vi "RT Driver VI.vi"(7 "Operation":T1, 11 "Device Reference in":T2 format="%.0x") -> (0 "Error Code":i32)   [LabVIEW 2021, in "Large Number Operation Engine.lvlib"]
uses:
  Large Number Operation Engine.lvlib
  <vilib>/NI VeriStand/Custom Device API/Custom Device Item Ref.ctl
  <vilib>/NI VeriStand/Custom Device API/Hardware Interface Driver VI Operation.ctl
  Shared/Compiled.Settings.ctl
  RTStateVariables.ctl
  <vilib>/NI/NIVS Inline Async API/_VS Inline Async API/VS Inline Async API/VS Inline Async API.lvclass
  <vilib>/NI/NIVS Inline Async API/_VS Inline Async API/VS Inline Async API/VS Inline Async API.lvclass/VS Inline Async API.ctl
  <vilib>/NI/NIVS Inline Async API/_Data Access Engine/Data Access Engine/Data Access Engine.lvclass/Data Access Engine.ctl
  <vilib>/NI/NIVS Inline Async API/_Data Access Engine/Access Type Classes/Write/Write.lvclass/Write.ctl
  <vilib>/NI/NIVS Inline Async API/_Data Access Engine/Access Type Classes/ReadWrite/ReadWrite.lvclass/ReadWrite.ctl
  <vilib>/NI/NIVS Inline Async API/_Data Access Engine/Access Type Classes/Read/Read.lvclass/Read.ctl
  <vilib>/NI/NIVS Inline Async API/_Data Access Engine/Data Access Engine/Methods/Data.Engine.Read Data from HW.vi
  <vilib>/NI/NIVS Inline Async API/_VS Inline Async API/Error Handling Process/SubVIs/Error.GetError.vi
  <vilib>/NI/NIVS Inline Async API/_Data Access Engine/Data Access Engine/Methods/Data.Engine.Write Data to HW.vi
  <vilib>/NI/NIVS Inline Async API/_Data Access Engine/Access Type Classes/ReadWrite/ReadWrite.EngineData.vi
  <vilib>/NI/NIVS Inline Async API/_Data Access Engine/Access Type Classes/Write/Write.EngineData.vi
  <vilib>/NI/NIVS Inline Async API/_Data Access Engine/Access Type Classes/Read/Read.EngineData.vi
  <vilib>/NI VeriStand/Custom Device API/NI VeriStand - Get Channel Value by Data Reference.vi
  <vilib>/NI VeriStand/Custom Device API/NI VeriStand - Set Channel Value by Data Reference.vi
  <vilib>/NI VeriStand/Custom Device API/NI VeriStand - Get Channel Values by Block Data Reference.vi
  Large Number Operation.Async.vi
  Shared/Constants.vi
  <vilib>/NI VeriStand/Custom Device API/Get Item Property (Variant).vi
  <vilib>/NI VeriStand/Custom Device API/Global Data Refs.vi
  <vilib>/NI VeriStand/Custom Device API/Custom Device API.lvlib
  Shared/Large Number Operation Shared.lvlib
  <vilib>/NI VeriStand/Custom Device Tools/Custom Device Utility Library/Custom Device Utility Library.lvlib
panel:
  out "appended array":cluster{"VI":refnum<vi>, "Parameters":variant}[](array[cluster])
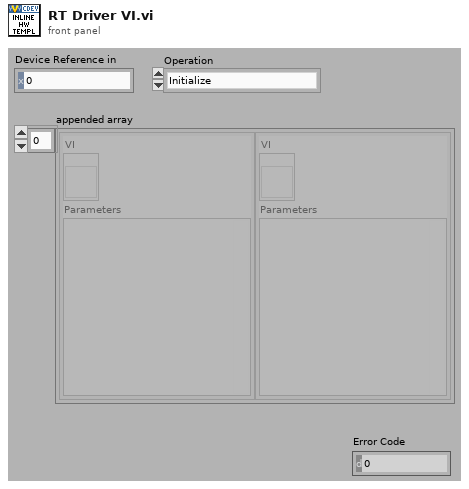
[diagram p1: front panel]
types:
  T1 = typedef "Custom Device API.lvlib/Hardware Interface Driver VI Operation.ctl" = enum16{"Initialize", "Start", "Read Data from HW", "Write Data to HW", "Close"}
  T2 = typedef "Custom Device API.lvlib/Custom Device Item Ref.ctl" = u64
  T3 = typedef "Large Number Operation Engine.lvlib/RTStateVariables.ctl" = cluster{"Async":refnum<class "VS Inline Async API.lvclass">, "Settings":T4}
  T4 = typedef "Large Number Operation Shared.lvlib/Compiled.Settings.ctl" = cluster{"Name":string, "Async Init Timeout":u16, "Address":string}
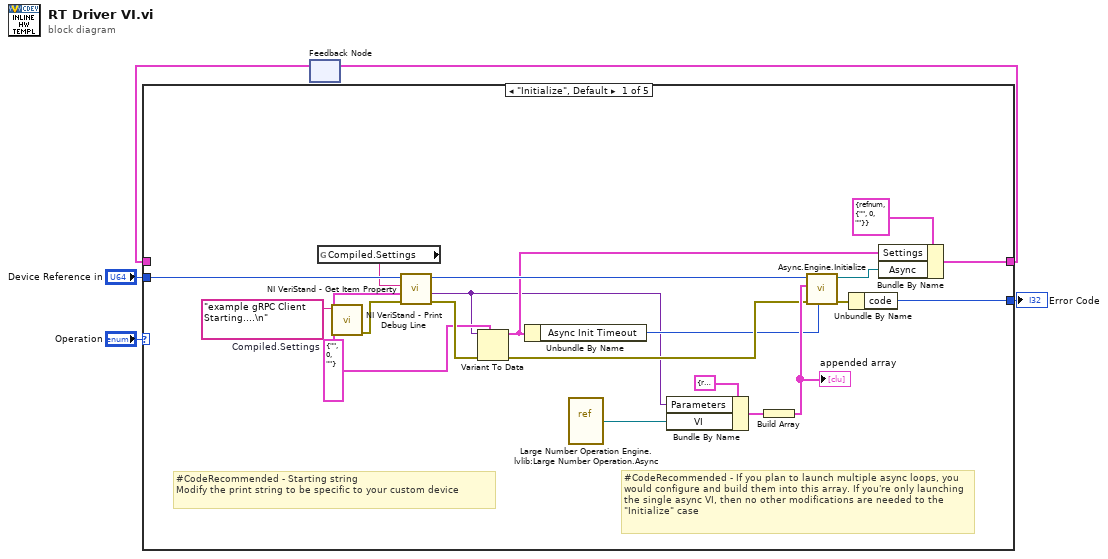
[diagram p0: block diagram]
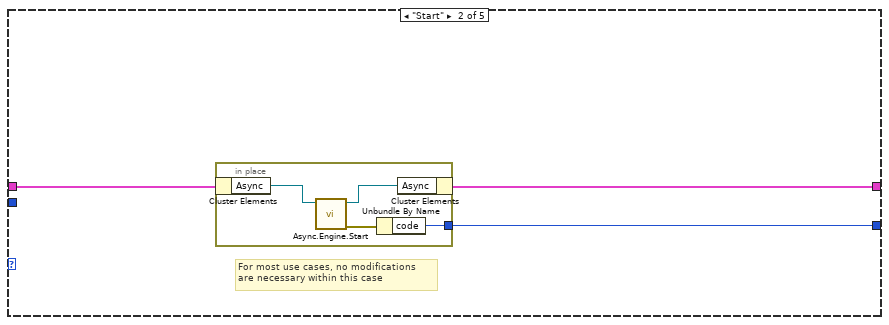
[diagram p2: hidden frame]
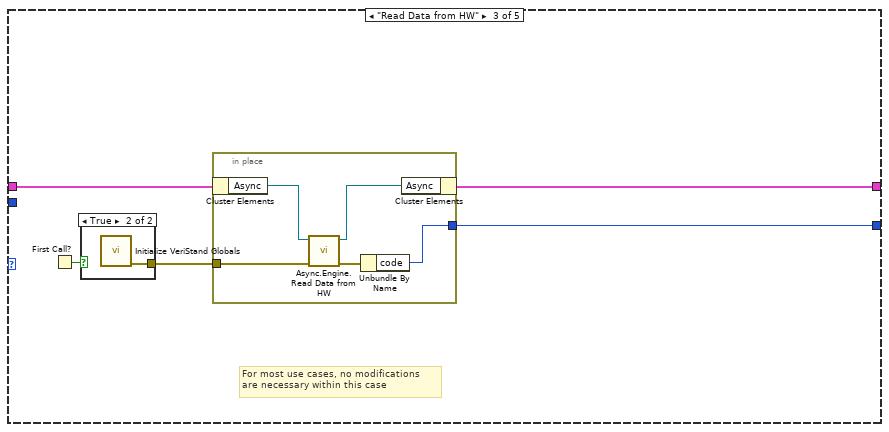
[diagram p3: hidden frame]
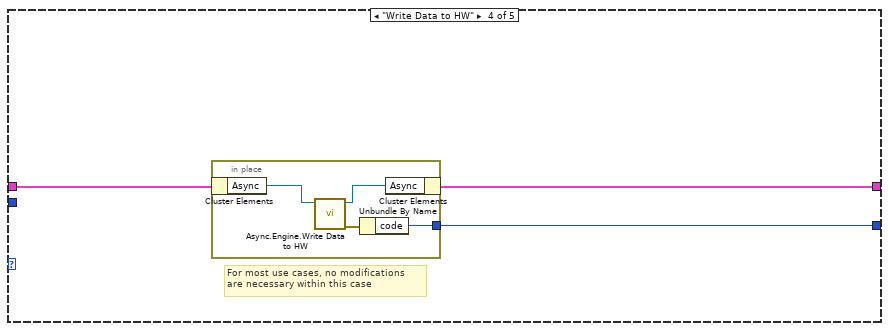
[diagram p5: hidden frame]
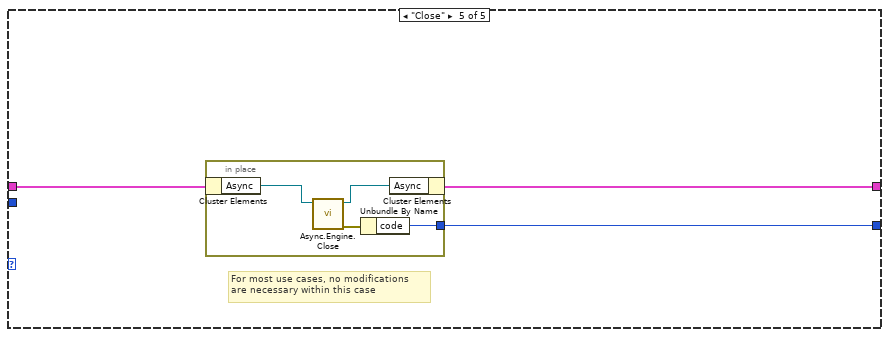
[diagram p6: hidden frame]
diagram:
  n1 = feedback #1() -> (w3:T3)  [unwired: 1 out]
  n2 = case shown="\"Initialize\", Default" "Operation" {
    tunnel: [w23 w27 w35 w44 w52] -> w4
    tunnel: w3 -> [_ w28 w37 w45 w53]
    tunnel: "Device Reference in" -> [w20 _ _ _ _]
    tunnel: [w25 w26 w36 w46 w51] -> w1
    frame "Initialize", Default {
      w16 = T4 {"Name"="", "Async Init Timeout"=0, "Address"=""}  # Compiled.Settings
      # "#CodeRecommended - Starting string\nModify the print string to be specific to your custom device"
      # "#CodeRecommended - If you plan to launch multiple async loops, you would configure and build them into this array. If you're only launching the single async VI, then no other modifications are needed to the \"Initialize\" case"
      n3 = global read "Constants.vi" "Compiled.Settings"() -> (w18:string)
      n4 = call <vilib>:"NI VeriStand - Print Debug Line.vi"("Message"="example gRPC Client Starting....\n") -> ("error out"=w12:errorcluster)  [unwired: 10 in]
      n5 = call-poly <vilib>:"NI VeriStand - Get Item Property.vi"("error in (no error)"=w12, "Default Value"=w16, "Property Name"=w18, "Item Ref in"=w20) -> ("error out"=w19:errorcluster, "Value"=w7:variant, "Item Ref out"=w13:T2)  [unwired: 4 in, 1 out]
      n6 = Variant To Data(error in=w19, type=w16, Variant=w7) -> (data=w8:T4, error out=w14:errorcluster)
      n7 = Unbundle By Name(w8) -> ("Async Init Timeout"=w9:u16)
      n8 = vi-ref "Large Number Operation Engine.lvlib:Large Number Operation.Async.vi"() -> (w10:refnum<vi>)
      n9 = Bundle By Name(cluster=cluster{"VI":refnum<vi>, "Parameters":variant} {"VI"=refnum, "Parameters"=variant} ("Process"), "Parameters"=w7, "VI"=w10) -> (w21:cluster{"VI":refnum<vi>, "Parameters":variant})
      n10 = Build Array(w21) -> (w15:cluster{"VI":refnum<vi>, "Parameters":variant}[])
      "appended array" <- w15
      n11 = call <vilib>:"Async.Engine.Initialize.vi"("Timeout (ms) (5000)"=w9, "error in (no error)"=w14, "Processes"=w15, "Custom Device Ref"=w13) -> ("error out"=w17:errorcluster, "Async"=w24:refnum<class "VS Inline Async API.lvclass">)  [unwired: 6 in]
      n12 = Unbundle By Name(w17) -> ("code"=w25:i32)
      n13 = Bundle By Name(cluster=T3 {"Async"=refnum, "Settings"={"Name"="", "Async Init Timeout"=0, "Address"=""}} ("RT State Variables"), "Settings"=w8, "Async"=w24) -> (w23:T3)
    }
    frame "Start" {
      # "For most use cases, no modifications \nare necessary within this case"
      n14 = in-place {
        in-place-border: [w29] -> w26
        n15 = in-place-cluster #2(w28) -> ("Async"=w32:refnum<class "VS Inline Async API.lvclass">)
        n16 = call <vilib>:"Async.Engine.Start.vi"("VS Inline Async API in"=w32) -> ("error out"=w30:errorcluster, "VS Inline Async API out"=w31:refnum<class "VS Inline Async API.lvclass">)  [unwired: 9 in]
        n17 = Unbundle By Name(w30) -> ("code"=w29:i32)
        n18 = in-place-cluster #2("Async"=w31) -> (w27:T3)
      }
    }
    frame "Read Data from HW" {
      # "For most use cases, no modifications \nare necessary within this case"
      n19 = First Call?() -> (First Call?: T/F=w33:bool)
      n20 = case shown="True" w33 {
        tunnel: [_ w38] -> w34
        frame False {
        }
        frame True {
          n21 = call "Initialize VeriStand Globals.vi"() -> ("error out"=w38:errorcluster)  [unwired: 11 in]
        }
      }
      n22 = in-place {
        in-place-border: [w41] -> w36
        in-place-border: w34 -> [w39]
        n23 = in-place-cluster #3(w37) -> ("Async"=w43:refnum<class "VS Inline Async API.lvclass">)
        n24 = call <vilib>:"Async.Engine.Read Data from HW.vi"("error in"=w39, "Async in"=w43) -> ("error out"=w40:errorcluster, "Async out"=w42:refnum<class "VS Inline Async API.lvclass">)  [unwired: 8 in]
        n25 = Unbundle By Name(w40) -> ("code"=w41:i32)
        n26 = in-place-cluster #3("Async"=w42) -> (w35:T3)
      }
    }
    frame "Write Data to HW" {
      # "For most use cases, no modifications \nare necessary within this case"
      n27 = in-place {
        in-place-border: [w50] -> w46
        n28 = in-place-cluster #4(w45) -> ("Async"=w48:refnum<class "VS Inline Async API.lvclass">)
        n29 = call <vilib>:"Async.Engine.Write Data to HW.vi"("VS Inline Async API in"=w48) -> ("error out"=w49:errorcluster, "VS Inline Async API out"=w47:refnum<class "VS Inline Async API.lvclass">)  [unwired: 9 in]
        n30 = Unbundle By Name(w49) -> ("code"=w50:i32)
        n31 = in-place-cluster #4("Async"=w47) -> (w44:T3)
      }
    }
    frame "Close" {
      # "For most use cases, no modifications \nare necessary within this case"
      n32 = in-place {
        in-place-border: [w55] -> w51
        n33 = in-place-cluster #5(w53) -> ("Async"=w57:refnum<class "VS Inline Async API.lvclass">)
        n34 = call <vilib>:"Async.Engine.Close.vi"("Async in"=w57) -> ("error out"=w54:errorcluster, "Async out"=w56:refnum<class "VS Inline Async API.lvclass">)  [unwired: 9 in]
        n35 = Unbundle By Name(w54) -> ("code"=w55:i32)
        n36 = in-place-cluster #5("Async"=w56) -> (w52:T3)
      }
    }
  }
  "Error Code" <- w1
  n37 = feedback-in #1(w4) -> ()
